vi "MakeDivArrayTwoBy.vi"(0 "B":T1={"Array Num"=[1, 2, 3], "Decimal Index"=0, "stop"=FALSE}) -> (1 "output array":cluster{"A":T1, "stop":bool}[](array[cluster]), 2 "Denom Info":cluster{"Denom":i32, "Offset":i32})   [LabVIEW 2025]
uses:
  Number.ctl
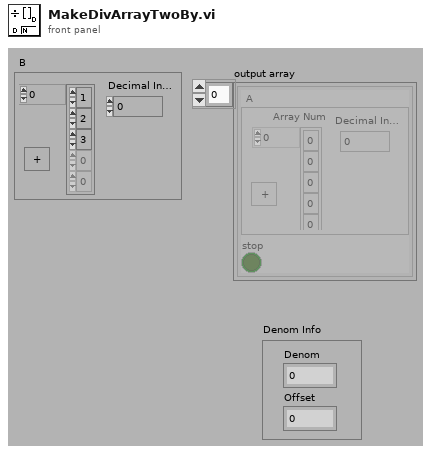
[diagram p1: front panel]
types:
  T1 = typedef "Number.ctl" = cluster{"Array Num":i8[], "Decimal Index":i32, "stop":bool}
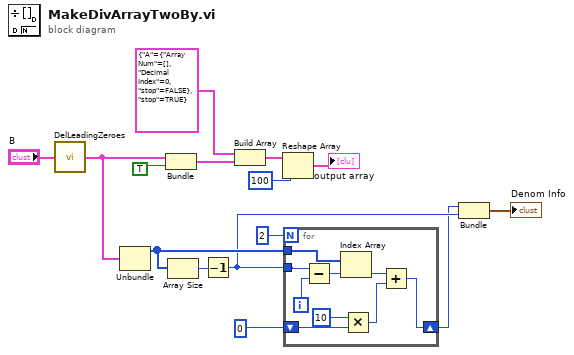
[diagram p0: block diagram]
diagram:
  n1 = call "DelLeadingZeroes.vi"("A 2"="B") -> ("A"=w3:T1)
  n2 = Unbundle(w3) -> ("Array Num"=w8:i8[])  [unwired: 2 out]
  n3 = Bundle("A"=w3, "stop"=TRUE) -> (w13:cluster{"A":T1, "stop":bool})  [unwired: 1 in]
  n4 = Array Size(array=w8) -> (size(s)=w9:i32)
  n5 = Decrement(x=w9) -> (x-1=w4:i32)
  n6 = Build Array(cluster{"A":T1, "stop":bool} {"A"={"Array Num"=[], "Decimal Index"=0, "stop"=FALSE}, "stop"=TRUE}, w13) -> (w11:cluster{"A":T1, "stop":bool}[])
  n7 = Reshape Array(w11, 100) -> (→"output array":cluster{"A":T1, "stop":bool}[])
  n8 = for {
    N: 2 ("f") -> [_]
    tunnel: w4 -> [w24]
    tunnel: w8 -> [w21]
    shift-right: [w16] -> w2
    shift-left: 0 ("f") -> [w18]
    i -> [w23]
    n9 = Subtract(x=w24, y=w23) -> (x-y=w22:i32)
    n10 = Index Array(array=w21, index=w22) -> (element=w20:i8)
    n11 = Multiply(x=10, y=w18) -> (x*y=w19:i32)
    n12 = Add(x=w20, y=w19) -> (x+y=w16:i32)
  }
  n13 = Bundle("f"=w2, w4) -> (→"Denom Info":cluster{"f":i32, i32})  [unwired: 1 in]
